vi "main.vi"() -> ()   [LabVIEW 2024]
uses:
  C:/Program Files (x86)/National Instruments/LabVIEW 2024/examples/Design Patterns/Queued Message Handler/support/QMH Fundamentals - Message Cluster.ctl
  isMapRun.vi
panel:
  in  "OK Button":bool
  out "display log":string
  in  "API key":string
  in  "Stop Button":bool
  in  "Start":bool
  out "Is Map running":bool
  in  "Tab Control":enum32{"Map", "Graph"}(tab)
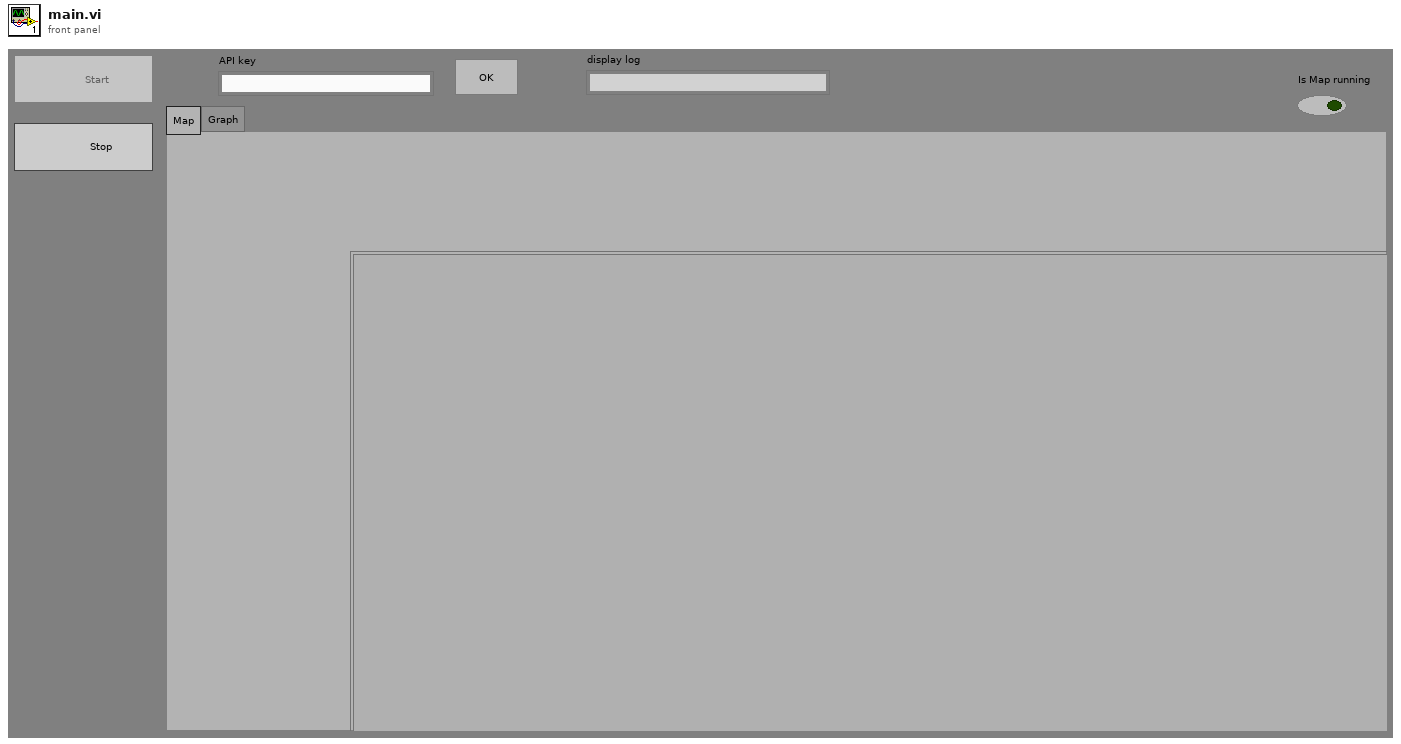
[diagram p1: front panel]
types:
  T1 = typedef "QMH Fundamentals - Message Cluster.ctl" = cluster{"Message":string, "Message Data":variant}
  T2 = enum16{"Always On", "Always Off", "Off While Running"}
  T3 = enum8{"Enabled", "Disabled", "Disabled and Grayed Out"}
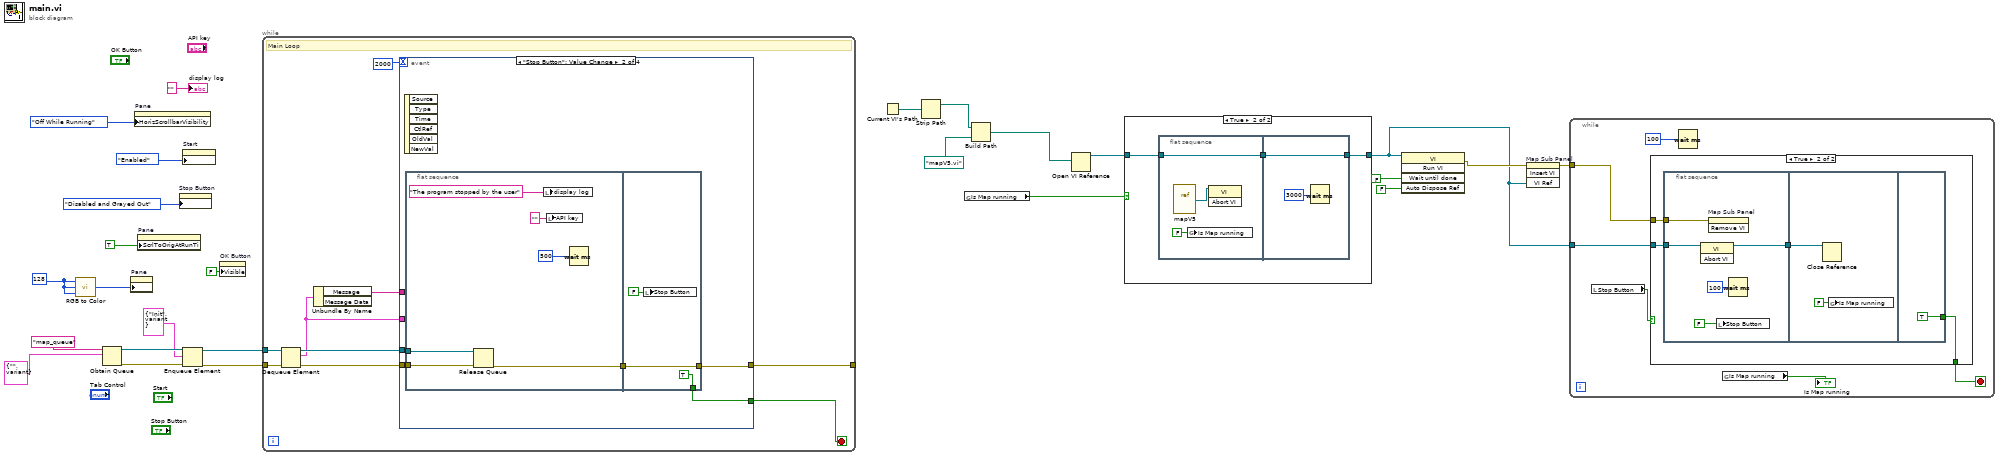
[diagram p0: block diagram]
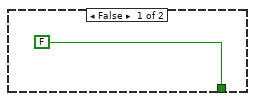
[diagram p3: hidden frame]
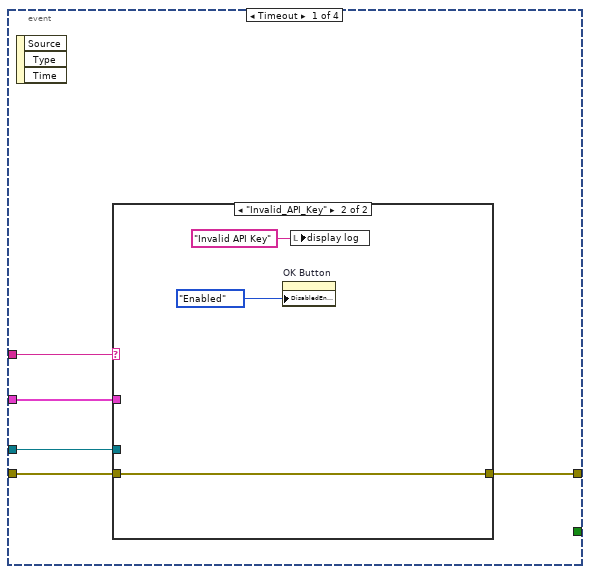
[diagram p4: hidden frame]
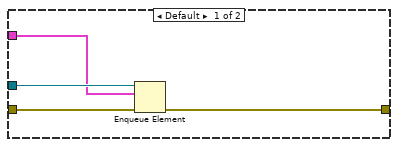
[diagram p5: hidden frame]
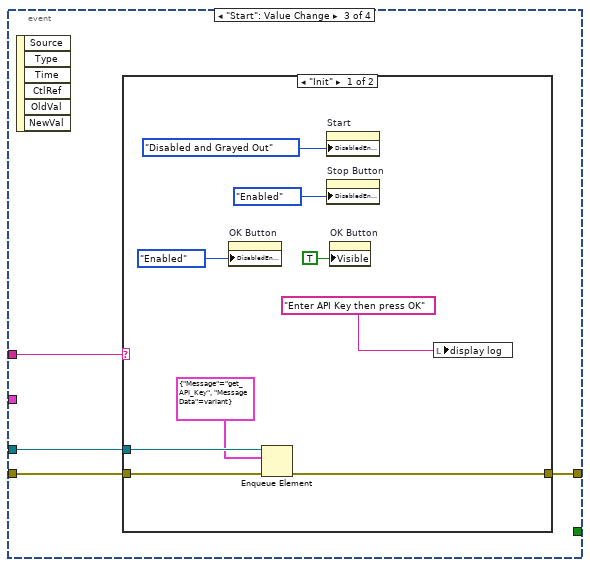
[diagram p6: hidden frame]
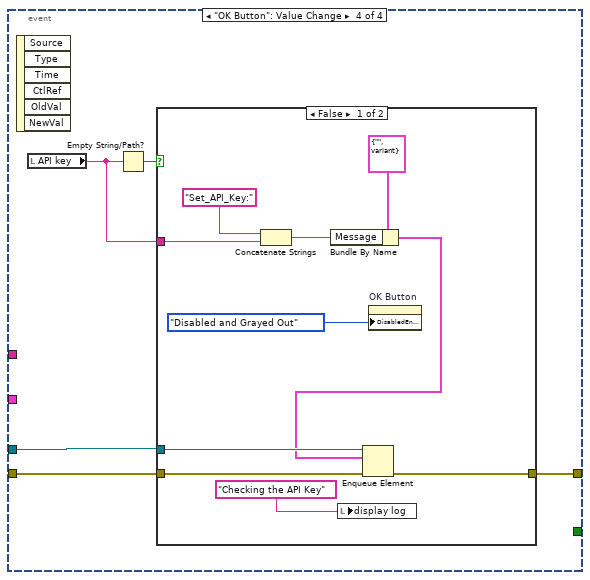
[diagram p8: hidden frame]
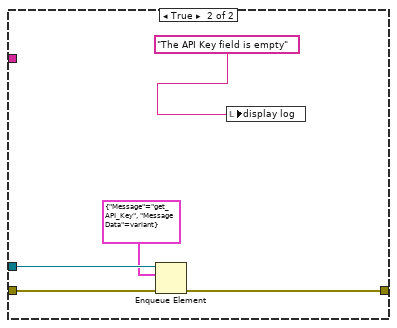
[diagram p9: hidden frame]
diagram:
  w22 = u8 128 ("R")
  n1 = call <vilib>:"RGB to Color.vi"("B"=w22, "G"=w22, "R"=w22) -> ("Color"=w23:u32)
  n2 = Obtain Queue(name (unnamed)="map_queue", element data type=T1 {"Message"="", "Message Data"=variant} ("Message Cluster")) -> (queue out=w17:refnum<queue>, error out=w15:errorcluster)  [unwired: 3 in, 1 out]
  n3 = property on="Pane" class="Pane"("PaneColor"=w23) -> ()  [unwired: 2 in, 2 out]
  n4 = property on="Pane" class="Pane"("HorizScrollbarVisibility"=T2."Off While Running" ("Horizontal Scrollbar Visibility")) -> ()  [unwired: 2 in, 2 out]
  n5 = property on="Pane" class="Pane"("ScrlToOrigAtRunTi"=TRUE ("Scroll To Origin At Run Time")) -> ()  [unwired: 2 in, 2 out]
  n6 = property on="Stop Button" class="Bool (strict)"("DisabledEnum"=T3."Disabled and Grayed Out" ("Disabled")) -> ()  [unwired: 2 in, 2 out]
  n7 = property on="Start" class="Bool"("DisabledEnum"=T3."Enabled" ("Disabled")) -> ()  [unwired: 2 in, 2 out]
  n8 = Enqueue Element(queue=w17, element=T1 {"Message"="Init", "Message Data"=variant}, error in (no error)=w15) -> (queue out=w14:refnum<queue>, error out=w13:errorcluster)  [unwired: 1 in, 1 out]
  n9 = property on="OK Button" class="Bool"("Visible"=FALSE) -> ()  [unwired: 2 in, 2 out]
  n10 = while {
    tunnel: w14 -> [w35]
    tunnel: w13 -> [w34]
    tunnel: [w30] -> _
    stop <- w27 stop-if-true
    # "Main Loop"
    n11 = Dequeue Element(queue=w35, error in (no error)=w34) -> (queue out=w32:refnum<queue>, element=w28:T1, error out=w31:errorcluster)  [unwired: 1 in, 1 out]
    n12 = Unbundle By Name(w28) -> ("Message"=w33:string)  [unwired: 1 out]
    n13 = event shown="[1] \"Stop Button\": Value Change" {
      selector: _ -> [_ _ _ _]
      dyn-events: _ -> [_ _ _ _]
      timeout: 2000 -> [_ _ _ _]
      tunnel: w33 -> [w40 _ w65 _]
      tunnel: w32 -> [w39 w51 w64 w77]
      tunnel: w31 -> [w38 w52 w63 w76]
      tunnel: [w36 w50 w62 w79] -> w30
      tunnel: w28 -> [w37 _ _ _]
      tunnel: [_ w48 _ _] -> w27
      event Timeout {
        n14 = event-data() -> ()  [unwired: 1 in, 3 out]
        n15 = case shown="\"Invalid_API_Key\"" w40 {
          tunnel: w39 -> [w44 _]
          tunnel: w38 -> [w43 w45]
          tunnel: w37 -> [w42 _]
          tunnel: [w41 w45] -> w36
          frame Default {
            n16 = Enqueue Element(queue=w44, element=w42, error in (no error)=w43) -> (error out=w41:errorcluster)  [unwired: 1 in, 2 out]
          }
          frame "Invalid_API_Key" {
            n17 = property on="OK Button" class="Bool"("DisabledEnum"=T3."Enabled" ("Disabled")) -> ()  [unwired: 2 in, 2 out]
            n18 = local write "display log"("Invalid API Key" ("display log")) -> ()
          }
        }
      }
      event "Stop Button": Value Change {
        n19 = event-data() -> ()  [unwired: 1 in, 6 out]
        n20 = flat-sequence {
          tunnel: w52 -> [w58]
          tunnel: w51 -> [w57]
          tunnel: [w56] -> w49
          tunnel: [w61] -> w50
          tunnel: w49 -> [w61]
          tunnel: [TRUE] -> w48
          frame #0 {
            n21 = Release Queue(queue=w57, error in (no error)=w58) -> (error out=w56:errorcluster)  [unwired: 1 in, 2 out]
            n22 = local write "display log"("The program stopped by the user" ("display log")) -> ()
            n23 = local write "API key"("" ("API key")) -> ()
            n24 = Wait (ms)(milliseconds to wait=u32 500) -> ()  [unwired: 1 out]
          }
          frame #1 {
            n25 = local write "Stop Button"(FALSE ("Stop Button")) -> ()
          }
        }
      }
      event "Start": Value Change {
        n26 = event-data() -> ()  [unwired: 1 in, 6 out]
        n27 = case shown="\"Init\"" w65 {
          tunnel: w64 -> [w71 _]
          tunnel: w63 -> [w70 w75]
          tunnel: [w68 w75] -> w62
          frame "Init" {
            n28 = property on="OK Button" class="Bool"("DisabledEnum"=T3."Enabled" ("Disabled")) -> ()  [unwired: 2 in, 2 out]
            n29 = Enqueue Element(queue=w71, element=T1 {"Message"="get_API_Key", "Message Data"=variant}, error in (no error)=w70) -> (error out=w68:errorcluster)  [unwired: 1 in, 2 out]
            n30 = property on="Start" class="Bool"("DisabledEnum"=T3."Disabled and Grayed Out" ("Disabled")) -> ()  [unwired: 2 in, 2 out]
            n31 = property on="Stop Button" class="Bool (strict)"("DisabledEnum"=T3."Enabled" ("Disabled")) -> ()  [unwired: 2 in, 2 out]
            n32 = property on="OK Button" class="Bool"("Visible"=TRUE) -> ()  [unwired: 2 in, 2 out]
            n33 = local write "display log"("Enter API Key then press OK" ("display log")) -> ()
          }
          frame Default {
          }
        }
      }
      event "OK Button": Value Change {
        n34 = event-data() -> ()  [unwired: 1 in, 6 out]
        n35 = local read "API key"() -> (w78:string)
        n36 = Empty String/Path?(string/path=w78) -> (empty?=w80:bool)
        n37 = case shown="False" w80 {
          tunnel: w77 -> [w90 w94]
          tunnel: w76 -> [w89 w93]
          tunnel: [w88 w91] -> w79
          tunnel: w78 -> [w86 _]
          frame False {
            n38 = Concatenate Strings("Set_API_Key:" ("string"), w86) -> (w85:string)
            n39 = Bundle By Name(cluster=T1 {"Message"="", "Message Data"=variant} ("Message Cluster"), "Message"=w85) -> (w83:T1)
            n40 = local write "display log"("Checking the API Key" ("display log")) -> ()
            n41 = Enqueue Element(queue=w90, element=w83, error in (no error)=w89) -> (error out=w88:errorcluster)  [unwired: 1 in, 2 out]
            n42 = property on="OK Button" class="Bool"("DisabledEnum"=T3."Disabled and Grayed Out" ("Disabled")) -> ()  [unwired: 2 in, 2 out]
          }
          frame True {
            n43 = Enqueue Element(queue=w94, element=T1 {"Message"="get_API_Key", "Message Data"=variant}, error in (no error)=w93) -> (error out=w91:errorcluster)  [unwired: 1 in, 2 out]
            n44 = local write "display log"("The API Key field is empty" ("display log")) -> ()
          }
        }
      }
    }
  }
  n45 = Current VI's Path() -> (path=w2:path)
  n46 = Strip Path(path=w2) -> (stripped path=w1:path)  [unwired: 1 out]
  n47 = global read "isMapRun.vi" "Is Map running"() -> (w5:bool)
  n48 = Build Path(base path=w1, name or relative path=path "mapV5.vi") -> (appended path=w3:path)
  n49 = Open VI Reference(vi path=w3) -> (vi reference=w7:refnum<vi>)  [unwired: 5 in, 1 out]
  n50 = case shown="True" w5 {
    tunnel: [w96 w99] -> w6
    tunnel: w7 -> [w96 w98]
    frame False {
    }
    frame True {
      n51 = flat-sequence {
        tunnel: w98 -> [w100]
        tunnel: [w100] -> w97
        tunnel: [w104] -> w99
        tunnel: w97 -> [w104]
        frame #0 {
          n52 = vi-ref "mapV5.vi"() -> (w101:refnum<vi>)
          n53 = global write "isMapRun.vi" "Is Map running"(FALSE ("Is Map running")) -> ()
          n54 = invoke class="VI" method="Abort VI"(reference=w101) -> ()  [unwired: 2 in, 3 out]
        }
        frame #1 {
          n55 = Wait (ms)(milliseconds to wait=u32 3000) -> ()  [unwired: 1 out]
        }
      }
    }
  }
  n56 = invoke class="VI" method="Run VI"(reference=w6, "Wait until done"=FALSE ("Wait Until Done"), "Auto Dispose Ref"=FALSE ("Auto Dispose Reference")) -> (error out=w10:errorcluster)  [unwired: 2 in, 4 out]
  n57 = invoke on="Map Sub Panel" class="SubPnl" method="Insert VI"(error in=w10, "VI Ref"=w6) -> (error out=w8:errorcluster)  [unwired: 2 in, 3 out]
  n58 = while {
    tunnel: w8 -> [w108]
    tunnel: w6 -> [w107]
    stop <- w109 stop-if-true
    n59 = local read "Stop Button"() -> (w105:bool)
    n60 = case shown="True" w105 {
      tunnel: [FALSE w114] -> w109
      tunnel: w108 -> [_ w115]
      tunnel: w107 -> [_ w112]
      frame False {
      }
      frame True {
        n61 = flat-sequence {
          tunnel: w115 -> [w120]
          tunnel: w112 -> [w118]
          tunnel: [w117] -> w113
          tunnel: w113 -> [w122]
          tunnel: [TRUE] -> w114
          frame #0 {
            n62 = invoke class="VI" method="Abort VI"(reference=w118) -> (reference out=w117:refnum<vi>)  [unwired: 2 in, 2 out]
            n63 = invoke on="Map Sub Panel" class="SubPnl" method="Remove VI"(error in=w120) -> ()  [unwired: 2 in, 3 out]
            n64 = local write "Stop Button"(FALSE ("stop")) -> ()
            n65 = Wait (ms)(milliseconds to wait=u32 100) -> ()  [unwired: 1 out]
          }
          frame #1 {
            n66 = Close Reference(reference=w122) -> ()  [unwired: 1 in, 1 out]
            n67 = global write "isMapRun.vi" "Is Map running"(FALSE ("Is Map running")) -> ()
          }
          frame #2 {
          }
        }
      }
    }
    n68 = Wait (ms)(milliseconds to wait=u32 100) -> ()  [unwired: 1 out]
    n69 = global read "isMapRun.vi" "Is Map running"() -> (→"Is Map running":bool)
  }
  "display log" <- "" ("display log")
